vi "E13_Semaforo_case_array.vi"() -> (0 "R4":bool, 1 "A4":bool, 2 "V4":bool, 3 "R3":bool, 4 "A3":bool, 5 "V3":bool, 6 "R2":bool, 7 "A2":bool, 8 "V2":bool, 9 "R1":bool, 10 "A1":bool, 11 "V1":bool)   [LabVIEW 2020]
panel:
  out "Seq 2":i32
  in  "stop 2":bool
  in  "stop":bool
  out "Seq":i32
  # "Array with Arduino"
  # "Case"
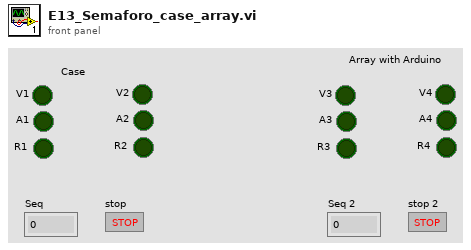
[diagram p1: front panel]
types:
  T1 = cluster{"[0]":bool, "[1]":bool, "[2]":bool, "[3]":bool, "[4]":bool, "[5]":bool, "[6]":bool, "[7]":bool, "[8]":bool}
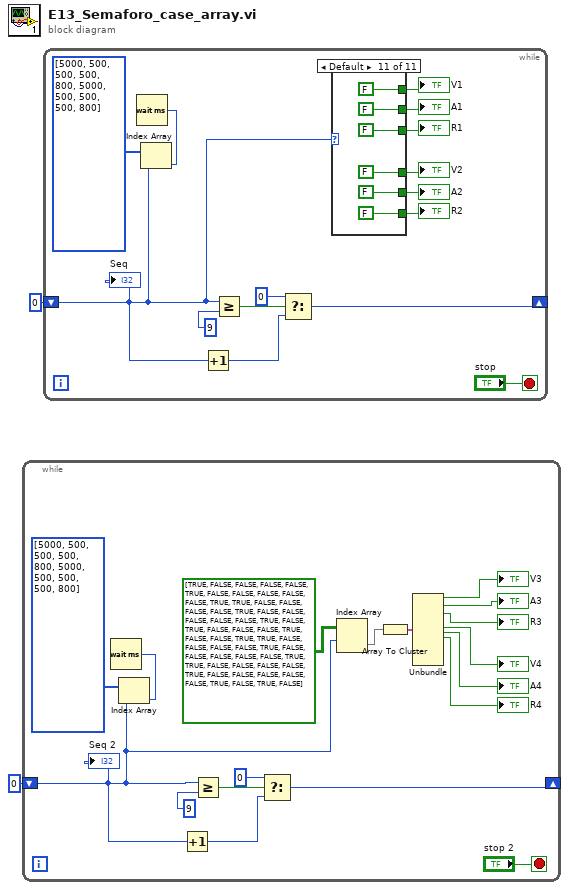
[diagram p0: block diagram]
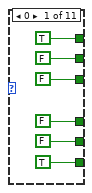
[diagram p2: hidden frame]
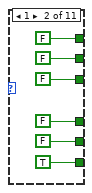
[diagram p3: hidden frame]
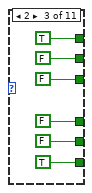
[diagram p4: hidden frame]
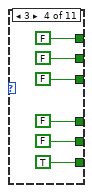
[diagram p5: hidden frame]
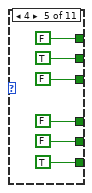
[diagram p6: hidden frame]
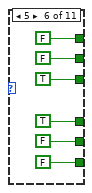
[diagram p7: hidden frame]
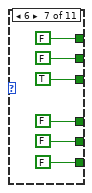
[diagram p8: hidden frame]
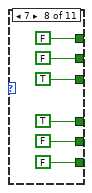
[diagram p9: hidden frame]
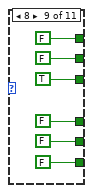
[diagram p10: hidden frame]
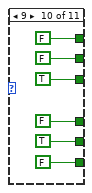
[diagram p11: hidden frame]
diagram:
  n1 = while {
    shift-right: [w19] -> _
    shift-left: 0 -> [w4]
    stop <- "stop 2" stop-if-true
    n2 = Index Array(array=u32[] [5000, 500, 500, 500, 800, 5000, 500, 500, 500, 800], index=w4) -> (element=w14:u32)
    n3 = Wait (ms)(milliseconds to wait=w14) -> ()  [unwired: 1 out]
    n4 = Increment(x=w4) -> (x+1=w18:i32)
    n5 = Greater Or Equal?(x=w4, y=9) -> (x >= y?=w20:bool)
    n6 = Select(t=0, s=w20, f=w18) -> (s? t:f=w19:i32)
    n7 = Index Array(array=bool[][] [[TRUE, FALSE, FALSE, FALSE, FALSE, TRUE], [FALSE, FALSE, FALSE, FALSE, FALSE, TRUE], [TRUE, FALSE, FALSE, FALSE, FALSE, TRUE], [FALSE, FALSE, FALSE, FALSE, FALSE, TRUE], [FALSE, TRUE, FALSE, FALSE, FALSE, TRUE], [FALSE, FALSE, TRUE, TRUE, FALSE, FALSE], [FALSE, FALSE, TRUE, FALSE, FALSE, FALSE], [FALSE, FALSE, TRUE, TRUE, FALSE, FALSE], [FALSE, FALSE, TRUE, FALSE, FALSE, FALSE], [FALSE, FALSE, TRUE, FALSE, TRUE, FALSE]], index (row)=w4) -> (element=w3:bool[])  [unwired: 1 in]
    n8 = Array To Cluster(array=w3) -> (cluster=w12:T1)
    n9 = Unbundle(w12) -> ("[0]"=→"V3":bool, "[1]"=→"A3":bool, "[2]"=→"R3":bool, "[3]"=→"V4":bool, "[4]"=→"A4":bool, "[5]"=→"R4":bool)  [unwired: 3 out]
    "Seq 2" <- w4
  }
  n10 = while {
    shift-right: [w34] -> _
    shift-left: 0 -> [w21]
    stop <- "stop" stop-if-true
    n11 = Index Array(array=u32[] [5000, 500, 500, 500, 800, 5000, 500, 500, 500, 800], index=w21) -> (element=w23:u32)
    n12 = Wait (ms)(milliseconds to wait=w23) -> ()  [unwired: 1 out]
    n13 = Increment(x=w21) -> (x+1=w33:i32)
    n14 = Greater Or Equal?(x=w21, y=9) -> (x >= y?=w35:bool)
    n15 = Select(t=0, s=w35, f=w33) -> (s? t:f=w34:i32)
    n16 = case shown="Default" w21 {
      tunnel: [TRUE FALSE TRUE FALSE FALSE FALSE FALSE FALSE FALSE FALSE FALSE] -> w30
      tunnel: [FALSE FALSE FALSE FALSE TRUE FALSE FALSE FALSE FALSE FALSE FALSE] -> w29
      tunnel: [FALSE FALSE FALSE FALSE FALSE TRUE TRUE TRUE TRUE TRUE FALSE] -> w28
      tunnel: [FALSE FALSE FALSE FALSE FALSE TRUE FALSE TRUE FALSE FALSE FALSE] -> w27
      tunnel: [FALSE FALSE FALSE FALSE FALSE FALSE FALSE FALSE FALSE TRUE FALSE] -> w26
      tunnel: [TRUE TRUE TRUE TRUE TRUE FALSE FALSE FALSE FALSE FALSE FALSE] -> w25
      frame 0 {
      }
      frame 1 {
      }
      frame 2 {
      }
      frame 3 {
      }
      frame 4 {
      }
      frame 5 {
      }
      frame 6 {
      }
      frame 7 {
      }
      frame 8 {
      }
      frame 9 {
      }
      frame Default {
      }
    }
    "V1" <- w30
    "A1" <- w29
    "R1" <- w28
    "V2" <- w27
    "A2" <- w26
    "R2" <- w25
    "Seq" <- w21
  }
